vi "TestInitializeOneShotSubscription_RejectOldValue.vi"(8 "error in (no error)":errorcluster, 11 "TestCase in":refnum<class "TestSubscriptionPolicy.lvclass">) -> (0 "error out":errorcluster, 3 "TestCase out":refnum<class "TestSubscriptionPolicy.lvclass">)   [LabVIEW 2017, in "TestSubscriptionPolicy.lvclass"]
uses:
  TestSubscriptionPolicy.lvclass
  gpm_packages/@cs/mva-core/Source/IMediator/ISubscriptionPolicy/ISubscriptionPolicy.lvclass
  gpm_packages/@cs/mva-core/Source/SubscriptionPolicy/OneShotSubscription/OneShotSubscription.lvclass
  gpm_packages/@cs/transport/Source/Concrete/QueueTransport/QueueTransport.lvclass
  C:/Git/mva-framework/gpm_packages/@cs/transport/Source/ITransport/ITransport.lvclass
  C:/Git/mva-framework/Source/Framework/IMediator/ISubscriptionPolicy/ISubscriptionPolicy.lvclass
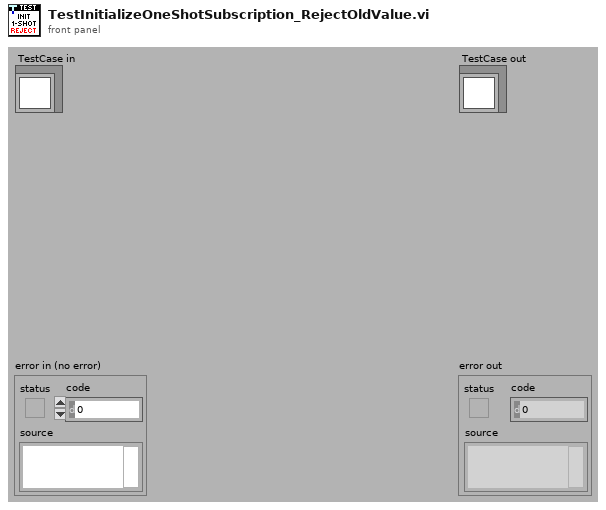
[diagram p1: front panel]
types:
  T1 = typedef "IMediator.lvlib/ISubscriptionPolicy.lvclass/ISubscriptionPolicy Reference.ctl" = refnum<data-value>
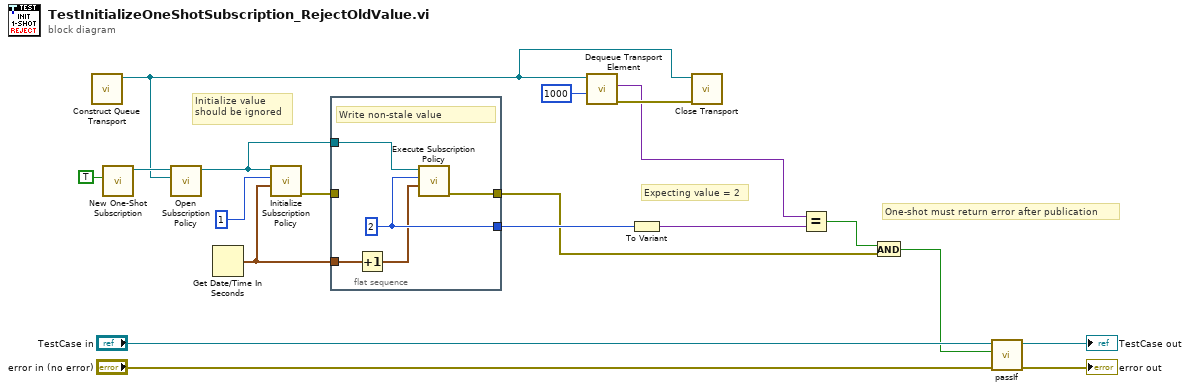
[diagram p0: block diagram]
diagram:
  # "Initialize value\nshould be ignored"
  # "One-shot must return error after publication"
  # "Expecting value = 2"
  n1 = call "Construct Queue Transport.vi"() -> ("QueueTransport"=w1:refnum<class "QueueTransport.lvclass">)  [unwired: 10 in, 1 out]
  n2 = call "New One-Shot Subscription.vi"("Ignore Past Updates? (F)"=TRUE) -> ("OneShotSubscription Out"=w13:refnum<class "OneShotSubscription.lvclass">)  [unwired: 10 in]
  n3 = call "Open Subscription Policy.vi"("Transport"=w1, "SubscriptionPolicy"=w13) -> ("Subscription Policy"=w6:T1)  [unwired: 8 in, 1 out]
  n4 = Get Date/Time In Seconds() -> (seconds since 1Jan1904=w4:timestamp)
  n5 = call "Initialize Subscription Policy.vi"("Last Publish Time"=w4, "Last Topic Value"=1, "Subscription Policy"=w6) -> ("Error Out (Unsubscribe?)"=w3:errorcluster)  [unwired: 7 in, 1 out]
  n6 = flat-sequence {
    tunnel: [w24] -> w11
    tunnel: [w23] -> w8
    tunnel: w6 -> [w22]
    tunnel: w4 -> [w21]
    tunnel: w3 -> [_]
    frame #0 {
      w24 = 2
      # "Write non-stale value"
      n7 = Increment(x=w21) -> (x+1=w20:timestamp)
      n8 = call "Execute Subscription Policy.vi"("Publish Time"=w20, "New Topic Value"=w24, "Subscription Policy"=w22) -> ("error out (Unsubscribe?)"=w23:errorcluster)  [unwired: 7 in, 1 out]
    }
  }
  n9 = call "Dequeue Transport Element.vi"("Timeout In ms (-1)"=1000, "QueueTransport"=w1) -> ("error out"=w14:errorcluster, "Data"=w2:variant)  [unwired: 6 in, 2 out]
  n10 = To Variant(anything=w11) -> (Variant=w10:variant)
  n11 = call-dynamic "Close Transport.vi"("error in (no error)"=w14, "QueueTransport"=w1) -> ()  [unwired: 9 in, 1 out]
  n12 = Equal?(x=w2, y=w10) -> (x = y?=w9:bool)
  n13 = And(x=w9, y=w8) -> (x .and. y?=w7:bool)
  n14 = call-dynamic "passIf.vi"("error in (no error)"="error in (no error)", "pass"=w7, "TestCase in"="TestCase in") -> ("error out"=→"error out":errorcluster, "TestCase out"=→"TestCase out":refnum<class "TestSubscriptionPolicy.lvclass">)  [unwired: 7 in]
